vi "DSF Configuration from JSON string.vi"(8 "error in (no error)":errorcluster, 10 "JSON string":string) -> (0 "error out":errorcluster, 3 "DSFConfiguration out":refnum<class "DSFConfiguration.lvclass">)   [LabVIEW 2017, in "DSFConfiguration.lvclass"]
uses:
  DSFConfiguration.lvclass
  Controls/dsf configuration file/1.0.0/dsf timing.ctl
  Controls/dsf configuration file/1.0.0/dsf configuration file v1.0.0.lvlib
  Controls/dsf configuration file/1.0.0/dsf plugin.ctl
  Controls/dsf configuration file/1.0.0/dsf group.ctl
  Controls/dsf configuration file/1.0.0/dsf transfer.ctl
  Controls/dsf configuration file/1.0.0/dsf channel.ctl
  Controls/dsf configuration file/1.0.0/dsf settings.ctl
  Controls/dsf configuration file/1.0.0/dsf configuration.ctl
  Controls/dsf configuration file/1.0.0/version.ctl
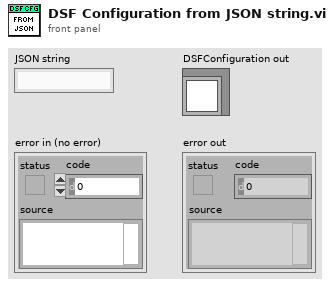
[diagram p1: front panel]
types:
  T1 = typedef "dsf configuration file v1.0.0.lvlib/dsf configuration.ctl" = cluster{"dsf schema version":T2, "configuration version":T2, "plugins":cluster{"id":string, "values":T3}[], "groups":cluster{"id":string, "values":T5}[], "transfers":cluster{"id":string, "values":T6}[], "channels":cluster{"id":string, "values":T7}[], "settings":cluster{"id":string, "values":T8}[]}
  T2 = typedef "dsf configuration file v1.0.0.lvlib/version.ctl" = cluster{"major":u32, "minor":u32, "fix":u32, "build":string}
  T3 = typedef "dsf configuration file v1.0.0.lvlib/dsf plugin.ctl" = cluster{"type":string, "timing":T4, "group ids":string[], "settings id":string}
  T4 = typedef "dsf configuration file v1.0.0.lvlib/dsf timing.ctl" = cluster{"decimation":i32, "offset":i32}
  T5 = typedef "dsf configuration file v1.0.0.lvlib/dsf group.ctl" = cluster{"direction":i32, "timing":T4, "transfer ids":string[], "settings id":string}
  T6 = typedef "dsf configuration file v1.0.0.lvlib/dsf transfer.ctl" = cluster{"byte order":i32, "channel ids":string[], "settings id":string}
  T7 = typedef "dsf configuration file v1.0.0.lvlib/dsf channel.ctl" = cluster{"count":i32, "offset":i32, "data type":dbl, "resource path":string, "settings id":string}
  T8 = typedef "dsf configuration file v1.0.0.lvlib/dsf settings.ctl" = cluster{"key":string, "value":string}[]
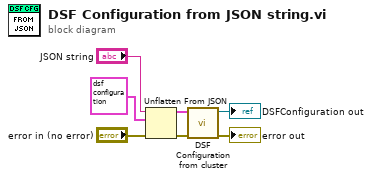
[diagram p0: block diagram]
diagram:
  n1 = Unflatten From JSON(JSON string="JSON string", type and defaults=T1 {"dsf schema version"={"major"=0, "minor"=0, "fix"=0, "build"=""}, "configuration version"={"major"=0, "minor"=0, "fix"=0, "build"=""}, "plugins"=[], "groups"=[], "transfers"=[], "channels"=[], "settings"=[]} ("configuration cluster"), error in (no error)="error in (no error)") -> (value=w1:T1, error out=w4:errorcluster)  [unwired: 4 in]
  n2 = call "DSF Configuration from cluster.vi"("error in (no error)"=w4, "configuration cluster"=w1) -> ("error out"=→"error out":errorcluster, "DSFConfiguration out"=→"DSFConfiguration out":refnum<class "DSFConfiguration.lvclass">)  [unwired: 8 in]
